vi "New Paragraph.vi"(7 "xwpfParagraph Type":refnum<class "xwpfParagraph.lvclass">, 8 "error in (no error)":errorcluster, 9 "Paragraph.Style":refnum<class "Style.lvclass">, 10 "Paragraph.Text":string, 11 "Paragraph.Ref":refnum<k24>) -> (0 "error out":errorcluster, 3 "xwpfParagraph out":refnum<class "xwpfParagraph.lvclass">)   [LabVIEW 2017, in "Word_Specific.lvlib" / "xwpfParagraph.lvclass"]
uses:
  xwpfParagraph.lvclass
  C:/Users/Neo/Desktop/Dev_Tools_BR/LabVIEW_NPOI/src/lib/NPOI 2.1.1/NPOI.OOXML.dll
  lib/NPOI 2.1.1/NPOI.OOXML.dll
  Styles/Style/Style.lvclass
  xwpfParagraph.lvclass/xwpfParagraph.ctl
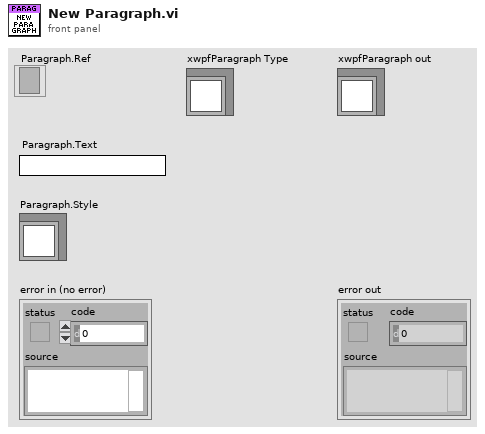
[diagram p1: front panel]
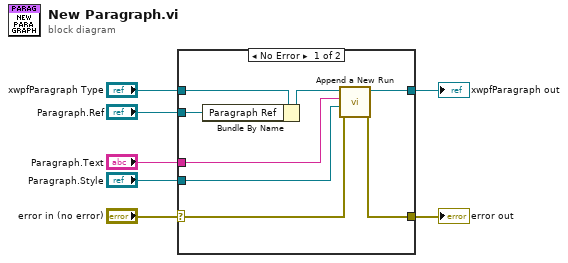
[diagram p0: block diagram]
diagram:
  n1 = case shown="No Error" "error in (no error)" {
    selector: "error in (no error)" -> [w11 w17]
    tunnel: [w14 w17] -> w6
    tunnel: [w15 w16] -> w4
    tunnel: "xwpfParagraph Type" -> [w10 w16]
    tunnel: "Paragraph.Ref" -> [w8 _]
    tunnel: "Paragraph.Style" -> [w13 _]
    tunnel: "Paragraph.Text" -> [w12 _]
    frame No Error {
      n2 = Bundle By Name(cluster=w10, "Paragraph Ref"=w8) -> (w9:refnum<class "xwpfParagraph.lvclass">)
      n3 = call "Append a New Run.vi"("error in (no error)"=w11, "Style"=w13, "Text"=w12, "xwpfParagraph in"=w9) -> ("error out"=w14:errorcluster, "xwpfParagraph out"=w15:refnum<class "xwpfParagraph.lvclass">)  [unwired: 6 in]
    }
    frame Error {
    }
  }
  "error out" <- w6
  "xwpfParagraph out" <- w4
